vi "Cleanup.vi"(8 "error in (no error)":errorcluster, 11 "Serial Stream in":refnum<class "Serial Stream.lvclass">) -> (0 "error out":errorcluster, 3 "Serial Stream out":refnum<class "Serial Stream.lvclass">)   [LabVIEW 2020, in "Stream-Serial.lvlib" / "Serial Stream.lvclass"]
uses:
  Serial Stream.lvclass
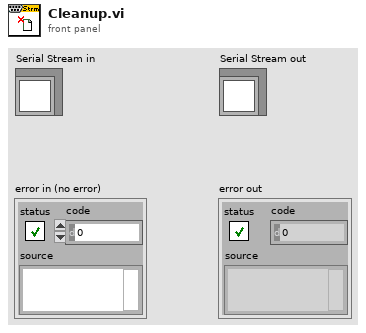
[diagram p1: front panel]
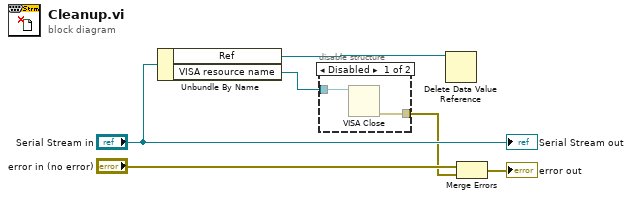
[diagram p0: block diagram]
diagram:
  n1 = Unbundle By Name("Serial Stream in") -> ("Ref"=w3:refnum<data-value>, "VISA resource name"=w4:refnum<visa-resource-name>)
  n2 = disable-structure shown="Disabled" {
    disable-tunnel: w4 -> [w8 _]
    disable-tunnel: [w7 _] -> w1
    frame Disabled {
      n3 = VISA Close(VISA resource name=w8) -> (error out=w7:errorcluster)  [unwired: 1 in]
    }
    frame Enabled {
    }
  }
  n4 = Delete Data Value Reference(data value reference=w3) -> ()  [unwired: 1 in, 2 out]
  n5 = Merge Errors("error in (no error)", w1) -> (→"error out":errorcluster)
  "Serial Stream out" <- "Serial Stream in"
